vi "has_[n]_solution.vi"(8 "error in (no error)":errorcluster, 11 "Instrument Command In":string) -> (0 "error out":errorcluster, 3 "Instrument Command In":string)   [LabVIEW 2018]
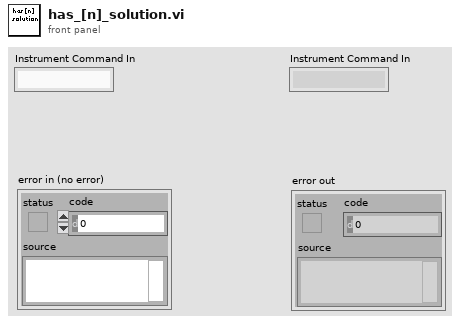
[diagram p1: front panel]
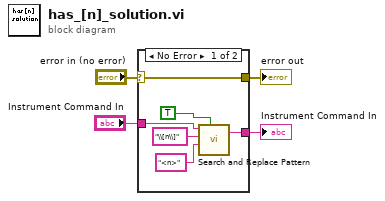
[diagram p0: block diagram]
diagram:
  n1 = case shown="No Error" "error in (no error)" {
    selector: "error in (no error)" -> [w5 w12]
    tunnel: "Instrument Command In" -> [w10 w11]
    tunnel: [w9 w11] -> w3
    tunnel: [w5 w12] -> w1
    frame No Error {
      n2 = call <vilib>:"Search and Replace Pattern.vi"("string"=w10, "regular expression (\"\")"="\\[n\\]" ("regular expression (\"\")"), "replace string (\"\")"="<n>" ("replace string (\"\")"), "replace all? (F)"=TRUE) -> ("result string"=w9:string)  [unwired: 2 out]
    }
    frame Error {
    }
  }
  "Instrument Command In" <- w3
  "error out" <- w1
